vi "PCU_Get_Device_ID.vi"(8 "error in (no error)":errorcluster) -> (0 "error out":errorcluster, 2 "id":string[](array[string]), 3 "Reference out":refnum<k24>)   [LabVIEW 2017]
uses:
  C:/Users/Ssantec_Test/Documents/GitHub/LV_Instrument_DLL_Sample/DLL/x86/InstrumentDLL.dll
  DLL/x86/InstrumentDLL.dll
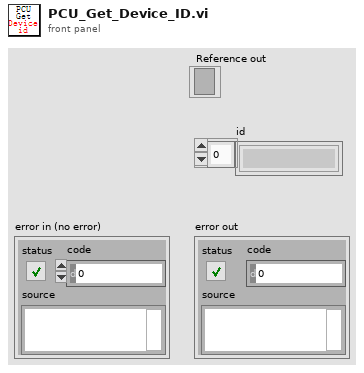
[diagram p1: front panel]
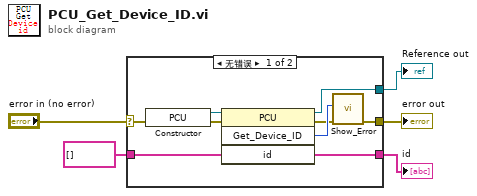
[diagram p0: block diagram]
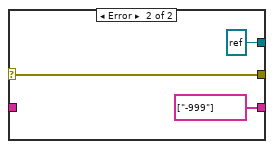
[diagram p2: hidden frame]
diagram:
  n1 = case shown="无错误" "error in (no error)" {
    selector: "error in (no error)" -> [w7 w17]
    tunnel: [w14 string[] ["-999"] ("id")] -> w5
    tunnel: string[] [] ("id") -> [w13 _]
    tunnel: [w12 refnum<k24> refnum ("new reference")] -> w3
    tunnel: [w9 w17] -> w2
    frame No Error {
      n2 = constructor class="PCU"(error in=w7) -> (reference out=w6:refnum<k24>, error out=w8:errorcluster)  [unwired: 2 in, 1 out]
      n3 = invoke on="调用节点" class="PCU" method="Get_Device_ID"(reference=w6, error in=w8, "id"=w13) -> (reference out=w12:refnum<k24>, error out=w10:errorcluster, "Get_Device_ID"=w11:i32, "id"=w14:string[])  [unwired: 1 in]
      n4 = call "Show_Error.vi"("error in (no error)"=w10, "Error"=w11) -> ("error out"=w9:errorcluster)  [unwired: 9 in]
    }
    frame Error {
    }
  }
  "id" <- w5
  "Reference out" <- w3
  "error out" <- w2
